vi "Save Graphic Overwrite.vi"(11 "Path":path) -> (2 "Cancel":bool, 3 "OK":bool)   [LabVIEW 2021]
uses:
  <resource>/plugins/NIIconEditor/Controls/IE Symbols.ctl
panel:
  in  "Symbol":T1=1
  out "String":string
  in  "string":string="This file already exists.\nDo you want to replace it?"
  in  "Cancel":bool
  in  "No":bool
  in  "Yes":bool
  out "error out":errorcluster
  in  "error in (no error)":errorcluster
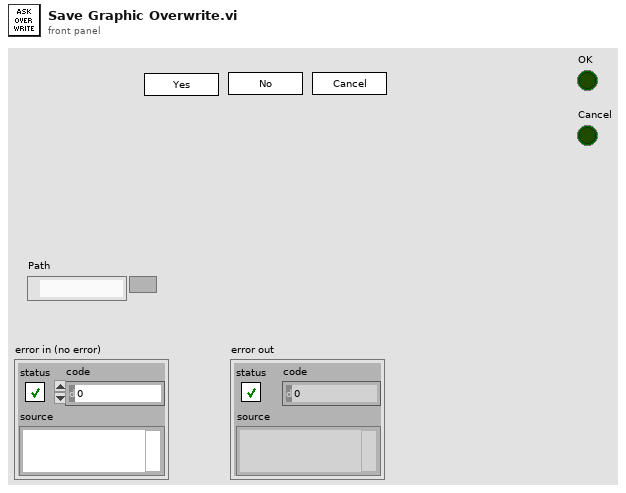
[diagram p1: front panel]
types:
  T1 = typedef "IE Symbols.ctl" = u16
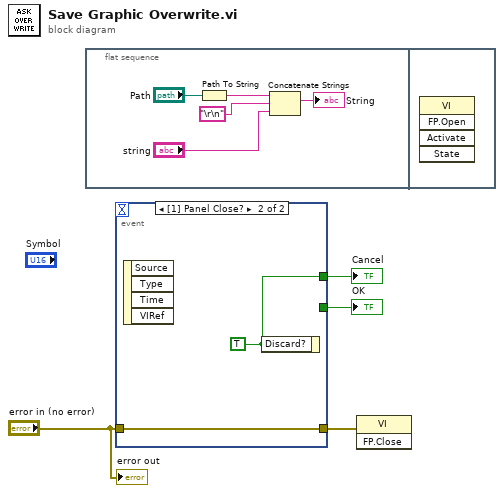
[diagram p0: block diagram]
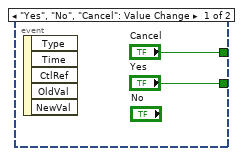
[diagram p2: hidden frame]
diagram:
  n1 = flat-sequence {
    frame #0 {
      n2 = Path To String(path="Path") -> (string=w8:string)
      n3 = Concatenate Strings(w8, "\r\n", "string") -> (→"String":string)
    }
    frame #1 {
      n4 = invoke class="VI" method="FP.Open"() -> ()  [unwired: 5 in, 5 out]
    }
  }
  n5 = event shown="[1] Panel Close?" {
    selector: _ -> [_ _]
    dyn-events: _ -> [_ _]
    timeout: _ -> [_ _]
    tunnel: ["Cancel" w13] -> w4
    tunnel: ["Yes" _] -> w3
    tunnel: [_ w12] -> w2
    tunnel: "error in (no error)" -> [_ w12]
    event "Yes", "No", "Cancel": Value Change {
      n6 = event-data() -> ()  [unwired: 1 in, 5 out]
    }
    event Panel Close? {
      w13 = TRUE ("Discard?")
      n7 = event-data() -> ()  [unwired: 1 in, 4 out]
      n8 = event-data("Discard?"=w13) -> ()  [unwired: 1 in, 1 out]
    }
  }
  "OK" <- w3
  "Cancel" <- w4
  n9 = invoke class="VI" method="FP.Close"(error in=w2) -> ()  [unwired: 2 in, 3 out]
  "error out" <- "error in (no error)"
